vi "OpenCVCam_Start.vi"(8 "ErrorIn":errorcluster, 10 "CmdData":variant, 11 "OpenCVCamIn":refnum<class>) -> (0 "ErrorOut":errorcluster, 2 "ReplyData":variant, 3 "OpenCVCamOut":refnum<class>, 4 "Exit":bool)   [LabVIEW 2021, in "OpenCVCam.lvclass"]
uses:
  OpenCVCam.lvclass
  OpenCVCam.lvclass/OpenCVCam.ctl
  State.ctl
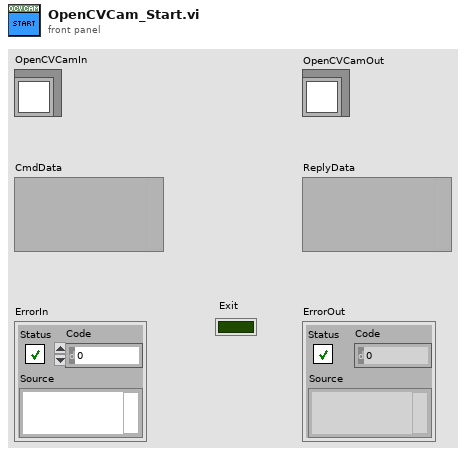
[diagram p1: front panel]
types:
  T1 = typedef "OpenCVCam.lvclass/State.ctl" = enum16{"Idle", "Initialized", "Acquiring"}
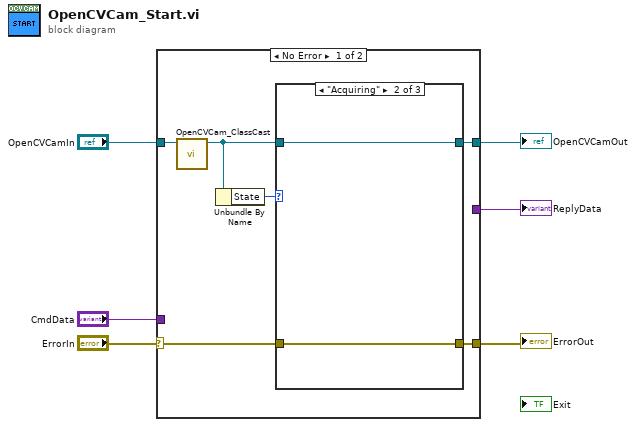
[diagram p0: block diagram]
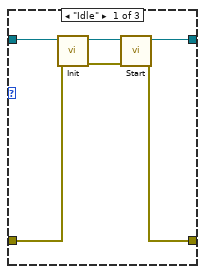
[diagram p2: hidden frame]
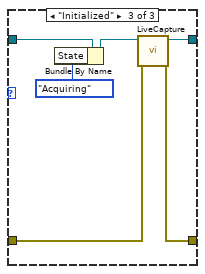
[diagram p3: hidden frame]
diagram:
  n1 = case shown="No Error" "ErrorIn" {
    selector: "ErrorIn" -> [w11 w29]
    tunnel: [w12 w29] -> w5
    tunnel: [_ w28] -> w3
    tunnel: "CmdData" -> [_ w28]
    tunnel: "OpenCVCamIn" -> [w10 w27]
    tunnel: [w9 w27] -> w1
    frame No Error {
      n2 = call "OpenCVCam_ClassCast.vi"("OpenCVCamIn"=w10) -> ("OpenCVCamOut"=w8:refnum<class "OpenCVCam.lvclass">)  [unwired: 10 in]
      n3 = Unbundle By Name(w8) -> ("State"=w7:T1)
      n4 = case shown="\"Acquiring\"" w7 {
        tunnel: [w13 w19 w24] -> w9
        tunnel: [w16 w20 w26] -> w12
        tunnel: w8 -> [w15 w19 w23]
        tunnel: w11 -> [w18 w20 w25]
        frame "Idle" {
          n5 = call-dynamic "Init.vi"("ErrorIn"=w18, "OpenCVCamIn"=w15) -> ("ErrorOut"=w17:errorcluster, "OpenCVCamOut"=w14:refnum<class "OpenCVCam.lvclass">)  [unwired: 8 in]
          n6 = call-dynamic "Start.vi"("ErrorIn"=w17, "OpenCVCamIn"=w14) -> ("ErrorOut"=w16:errorcluster, "OpenCVCamOut"=w13:refnum<class "OpenCVCam.lvclass">)  [unwired: 8 in]
        }
        frame "Acquiring" {
        }
        frame "Initialized" {
          n7 = Bundle By Name(cluster=w23, "State"=State."Acquiring" ("Local.State")) -> (w22:refnum<class "OpenCVCam.lvclass">)
          n8 = call-dynamic "LiveCapture.vi"("ErrorIn"=w25, "OpenCVCamIn"=w22) -> ("ErrorOut"=w26:errorcluster, "OpenCVCamOut"=w24:refnum<class "OpenCVCam.lvclass">)  [unwired: 8 in]
        }
      }
    }
    frame Error {
    }
  }
  "ErrorOut" <- w5
  "OpenCVCamOut" <- w1
  "ReplyData" <- w3
